vi "Command - Wave Control.vi"(0 "VISA Refnum in":refnum<visa-resource-name>, 1 "Value":dbl=2.0, 2 "Unit":string, 5 "Channel":i32, 7 "Command":T2(ring), 9 "Wave Type":T1(ring), 11 "Error In":errorcluster, 12 "Command Type":enum16{"Set", "Get"}(ring), 13 "Bytes to Read":u32) -> (4 "VISA Refnum out":refnum<visa-resource-name>, 6 "Read Buffer":string, 15 "Error Out":errorcluster)   [LabVIEW 2025]
panel:
  out "Command Out":string
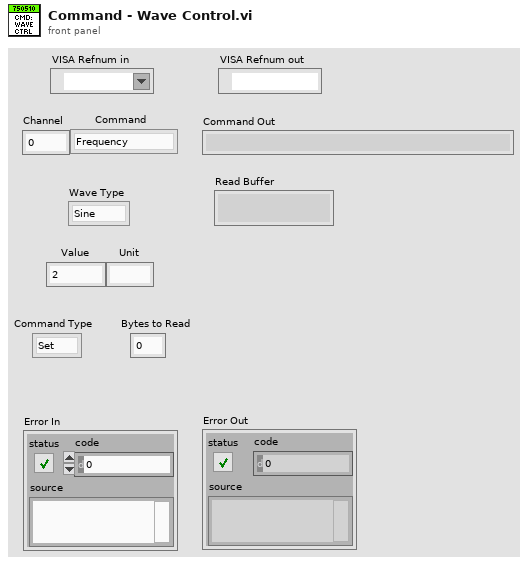
[diagram p1: front panel]
types:
  T1 = enum16{"Sine", "Square", "Triangle", "Pulse", "Built In"}
  T2 = enum16{"Frequency", "Voltage Level", "Voltage Offset", "Phase", "Phase Sync", "Wave Type"}
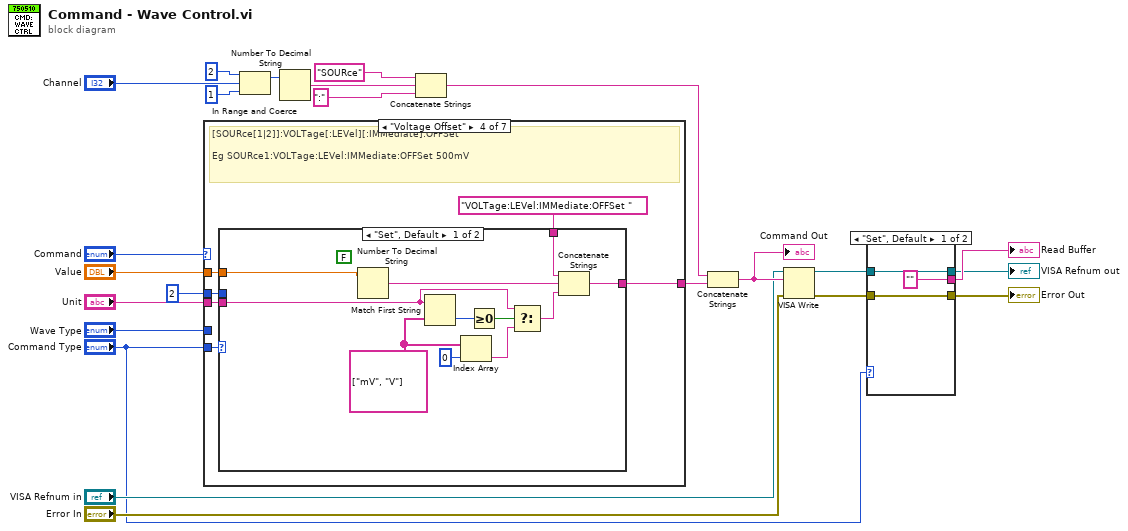
[diagram p0: block diagram]
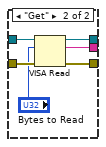
[diagram p2: hidden frame]
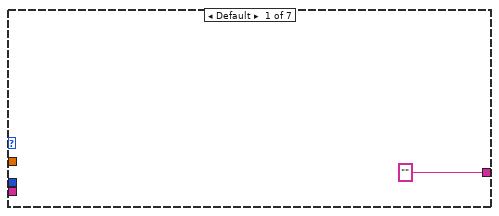
[diagram p3: hidden frame]
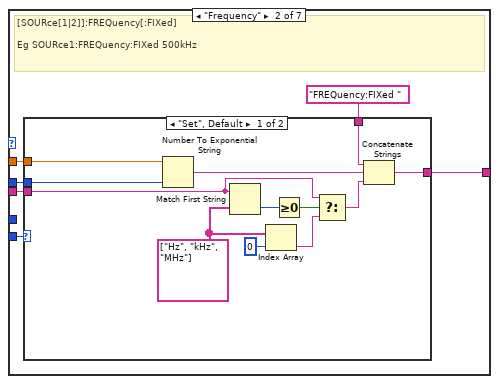
[diagram p4: hidden frame]
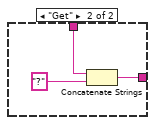
[diagram p5: hidden frame]
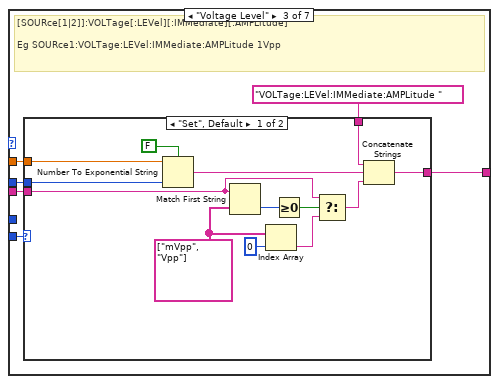
[diagram p6: hidden frame]
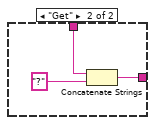
[diagram p7: hidden frame]
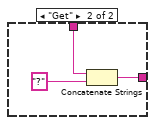
[diagram p8: hidden frame]
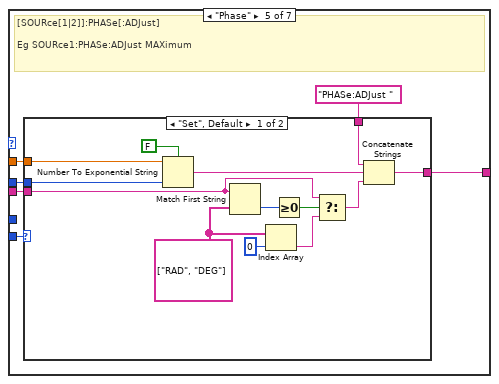
[diagram p9: hidden frame]
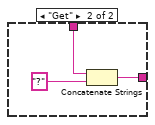
[diagram p10: hidden frame]
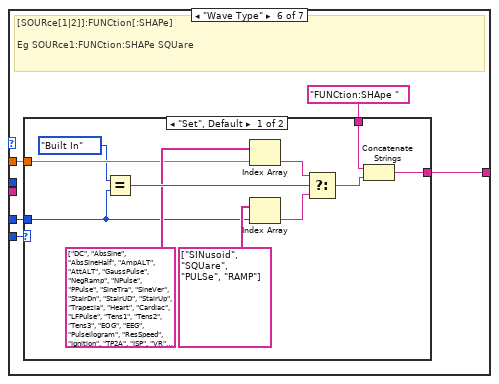
[diagram p11: hidden frame]
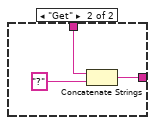
[diagram p12: hidden frame]
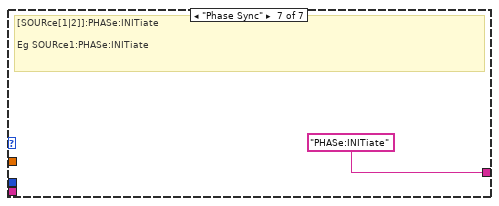
[diagram p13: hidden frame]
diagram:
  n1 = case shown="\"Voltage Offset\"" "Command" {
    tunnel: ["" w29 w50 w72 w92 w113 "PHASe:INITiate"] -> w20
    tunnel: "Value" -> [_ w28 w49 w71 w91 w112 _]
    tunnel: "Unit" -> [_ w27 w48 w70 w90 _ _]
    tunnel: "Wave Type" -> [_ _ _ _ _ w111 _]
    tunnel: "Command Type" -> [_ w26 w47 w69 w89 w110 _]
    tunnel: i16 2 ("precision (6)") -> [_ w25 w46 w68 w88 _ _]
    frame Default {
    }
    frame "Frequency" {
      # "[SOURce[1|2]]:FREQuency[:FIXed]\n\nEg SOURce1:FREQuency:FIXed 500kHz"
      n2 = case shown="\"Set\", Default" w26 {
        tunnel: "FREQuency:FIXed " -> [w42 w44]
        tunnel: [w41 w45] -> w29
        tunnel: w28 -> [w40 _]
        tunnel: w27 -> [w36 _]
        tunnel: w25 -> [w31 _]
        frame "Set", Default {
          w34 = string[] ["Hz", "kHz", "MHz"]
          n3 = Number To Exponential String(number=w40, precision (6)=w31) -> (E-format string=w39:string)  [unwired: 2 in]
          n4 = Match First String(2:w34, 3:w36) -> (0:w38:i32)  [unwired: 1 out]
          n5 = Index Array(array=w34, index=0) -> (element=w35:string)
          n6 = Greater Or Equal To 0?(x=w38) -> (x >= 0?=w37:bool)
          n7 = Select(t=w36, s=w37, f=w35) -> (s? t:f=w32:string)
          n8 = Concatenate Strings(w42, w39, w32) -> (w41:string)
        }
        frame "Get" {
          n9 = Concatenate Strings(w44, "?" ("string")) -> (w45:string)
        }
      }
    }
    frame "Voltage Level" {
      # "[SOURce[1|2]]:VOLTage[:LEVel][:IMMediate][:AMPLitude]\n\nEg SOURce1:VOLTage:LEVel:IMMediate:AMPLitude 1Vpp"
      n10 = case shown="\"Set\", Default" w47 {
        tunnel: "VOLTage:LEVel:IMMediate:AMPLitude " -> [w64 w65]
        tunnel: [w63 w66] -> w50
        tunnel: w49 -> [w62 _]
        tunnel: w48 -> [w58 _]
        tunnel: w46 -> [w52 _]
        frame "Set", Default {
          w56 = string[] ["mVpp", "Vpp"]
          n11 = Number To Exponential String(number=w62, precision (6)=w52, 1:FALSE ("use system decimal point (T)")) -> (E-format string=w61:string)  [unwired: 1 in]
          n12 = Match First String(2:w56, 3:w58) -> (0:w60:i32)  [unwired: 1 out]
          n13 = Index Array(array=w56, index=0) -> (element=w57:string)
          n14 = Greater Or Equal To 0?(x=w60) -> (x >= 0?=w59:bool)
          n15 = Select(t=w58, s=w59, f=w57) -> (s? t:f=w54:string)
          n16 = Concatenate Strings(w64, w61, w54) -> (w63:string)
        }
        frame "Get" {
          n17 = Concatenate Strings(w65, "?" ("string")) -> (w66:string)
        }
      }
    }
    frame "Voltage Offset" {
      # "[SOURce[1|2]]:VOLTage[:LEVel][:IMMediate]:OFFSet\n\nEg SOURce1:VOLTage:LEVel:IMMediate:OFFSet 500mV"
      n18 = case shown="\"Set\", Default" w69 {
        tunnel: "VOLTage:LEVel:IMMediate:OFFSet " -> [w84 w85]
        tunnel: [w83 w86] -> w72
        tunnel: w71 -> [w74 _]
        tunnel: w70 -> [w79 _]
        tunnel: w68 -> [_ _]
        frame "Set", Default {
          (unwired) FALSE ("use system decimal point (T)")
          w77 = string[] ["mV", "V"]
          n19 = Number To Decimal String(number=w74) -> (decimal integer string=w82:string)  [unwired: 1 in]
          n20 = Match First String(2:w77, 3:w79) -> (0:w81:i32)  [unwired: 1 out]
          n21 = Index Array(array=w77, index=0) -> (element=w78:string)
          n22 = Greater Or Equal To 0?(x=w81) -> (x >= 0?=w80:bool)
          n23 = Select(t=w79, s=w80, f=w78) -> (s? t:f=w75:string)
          n24 = Concatenate Strings(w84, w82, w75) -> (w83:string)
        }
        frame "Get" {
          n25 = Concatenate Strings(w85, "?" ("string")) -> (w86:string)
        }
      }
    }
    frame "Phase" {
      # "[SOURce[1|2]]:PHASe[:ADJust]\n\nEg SOURce1:PHASe:ADJust MAXimum"
      n26 = case shown="\"Set\", Default" w89 {
        tunnel: "PHASe:ADJust " -> [w106 w107]
        tunnel: [w105 w108] -> w92
        tunnel: w91 -> [w104 _]
        tunnel: w90 -> [w100 _]
        tunnel: w88 -> [w94 _]
        frame "Set", Default {
          w98 = string[] ["RAD", "DEG"]
          n27 = Number To Exponential String(number=w104, precision (6)=w94, 1:FALSE ("use system decimal point (T)")) -> (E-format string=w103:string)  [unwired: 1 in]
          n28 = Match First String(2:w98, 3:w100) -> (0:w102:i32)  [unwired: 1 out]
          n29 = Index Array(array=w98, index=0) -> (element=w99:string)
          n30 = Greater Or Equal To 0?(x=w102) -> (x >= 0?=w101:bool)
          n31 = Select(t=w100, s=w101, f=w99) -> (s? t:f=w96:string)
          n32 = Concatenate Strings(w106, w103, w96) -> (w105:string)
        }
        frame "Get" {
          n33 = Concatenate Strings(w107, "?" ("string")) -> (w108:string)
        }
      }
    }
    frame "Wave Type" {
      # "[SOURce[1|2]]:FUNCtion[:SHAPe]\n\nEg SOURce1:FUNCtion:SHAPe SQUare"
      n34 = case shown="\"Set\", Default" w110 {
        tunnel: "FUNCtion:SHApe " -> [w125 w126]
        tunnel: [w124 w127] -> w113
        tunnel: w112 -> [w120 _]
        tunnel: w111 -> [w119 _]
        frame "Set", Default {
          n35 = Equal?(x=T1."Built In" ("y"), y=w119) -> (x = y?=w122:bool)
          n36 = Index Array(array=string[] ["DC", "AbsSine", "AbsSineHalf", "AmpALT", "AttALT", "GaussPulse", "NegRamp", "NPulse", "PPulse", "SineTra", "SineVer", "StairDn", "StairUD", "StairUp", "Trapezia", "Heart", "Cardiac", "LFPulse", "Tens1", "Tens2", "Tens3", "EOG", "EEG", "Pulseilogram", "ResSpeed", "Ignition", "TP2A", "ISP", "VR", "TP1", "TP2B", "P4", "TP5A", "TP5B", "SCR", "Surge", "Airy", "Besselj", "Bessely", "Cauchy", "X^3", "Erf", "Erfc", "ErfcInv", "ErfInv", "Dirichlet", "ExpFall", "ExpRise", "Laguerre", "Laplace", "Legend", "Gauss", "HaverSine", "Log", "LogNormal", "Lorentz", "Maxwell", "Rayleigh", "Versiera", "Weibull", "Ln(x)", "X^2", "Round", "Chirp", "Rhombus", "CosH", "Cot", "CotH", "CotHCon", "CotHPro", "CscCon", "Csc", "CscPro", "CscH", "CscHCon", "CscHPro", "RecipCon", "RecipPro", "SecCon", "SecPro", "SecH", "Sinc", "SinH", "Sqrt", "Tan", "TanH", "ACos", "ACosH", "ACot", "ACotCon", "ACotPro", "ACotH", "ACotHCon", "ACotHPro", "Acsc", "ACscCon", "ACscPro", "AcscH", "ACscHCon", "ACscHPro", "Asec", "ASecCon", "ASecPro", "ASecH", "ASin", "ASinH", "ATan", "ATanH", "Bartlett", "BarthannWin", "Blackman", "BlackmanH", "BohmanWin", "Boxcar", "ChebWin", "FlattopWin", "Hamming", "Hanning", "Kaiser", "NuttallWin", "ParzenWin", "TaylorWin", "Triang", "TukeyWin", "Butterworth", "Combin", "CPulse", "CWPulse", "RoundHalf", "BandLimited", "BlaseiWave", "Chebyshev1", "Chebyshev2", "DampedOsc", "DualTone", "Gamma", "GateVibar", "LFMPulse", "MCNoise", "Discharge", "Quake", "Radar", "Ripple", "RoundsPM", "StepResp", "SwingOsc", "TV", "Voice", "AM", "FM", "PM", "PWM"] ("Array"), index=w120) -> (element=w117:string)
          n37 = Index Array(array=string[] ["SINusoid", "SQUare", "PULSe", "RAMP"], index=w119) -> (element=w116:string)
          n38 = Select(t=w117, s=w122, f=w116) -> (s? t:f=w115:string)
          n39 = Concatenate Strings(w125, w115) -> (w124:string)
        }
        frame "Get" {
          n40 = Concatenate Strings(w126, "?" ("string")) -> (w127:string)
        }
      }
    }
    frame "Phase Sync" {
      # "[SOURce[1|2]]:PHASe:INITiate\n\nEg SOURce1:PHASe:INITiate"
    }
  }
  n41 = In Range and Coerce(upper limit=2, x="Channel", lower limit=1) -> (coerced(x)=w15:i32)  [unwired: 1 out]
  n42 = Number To Decimal String(number=w15) -> (decimal integer string=w17:string)  [unwired: 1 in]
  n43 = Concatenate Strings("SOURce", w17, ":") -> (w21:string)
  n44 = Concatenate Strings(w21, w20) -> (w5:string)
  "Command Out" <- w5
  n45 = VISA Write(VISA resource name="VISA Refnum in", write buffer=w5, error in (no error)="Error In") -> (VISA resource name out=w6:refnum<visa-resource-name>, error out=w7:errorcluster)  [unwired: 1 out]
  n46 = case shown="\"Set\", Default" "Command Type" {
    tunnel: w6 -> [w131 w138]
    tunnel: w7 -> [w132 w137]
    tunnel: [w132 w136] -> w8
    tunnel: [w131 w135] -> w9
    tunnel: ["" ("read buffer") w134] -> w10
    frame "Set", Default {
    }
    frame "Get" {
      n47 = VISA Read(VISA resource name=w138, byte count="Bytes to Read", error in (no error)=w137) -> (VISA resource name out=w135:refnum<visa-resource-name>, read buffer=w134:string, error out=w136:errorcluster)  [unwired: 1 out]
    }
  }
  "Read Buffer" <- w10
  "VISA Refnum out" <- w9
  "Error Out" <- w8
